vi "INitTape.vi"(5 "Settings in":T1={"max velocity"={"Value"=0.0, "Min"=0.0, "Max"=0.0, "StepSize"=0.0, "Tolerance"=0.0, "valueactual"=0.0}, "continious velocity"={"Value"=0.0, "Min"=0.0, "Max"=0.0, "StepSize"=0.0, "Tolerance"=0.0, "valueactual"=0.0}, "shake"=enum."off", "direction"=enum."left", "RedRatio"={"Value"=0.0, "Min"=0.0, "Max"=0.0, "StepSize"=0.0, "Tolerance"=0.0, "valueactual"=0.0}, "StepSize"={"Value"=0.0, "Min"=0.0, "Max"=0.0, "StepSize"=0.0, "Tolerance"=0.0, "valueactual"=0.0}, "position"={"Value"=0.0, "Min"=0.0, "Max"=0.0, "StepSize"=0.0, "Tolerance"=0.0, "valueactual"=0.0}, "velocity"={"Value"=0.0, "Min"=0.0, "Max"=0.0, "StepSize"=0.0, "Tolerance"=0.0, "valueactual"=0.0}, "Step"=enum."off", "Mode"=enum."on demand", "timeout"={"Value"=0.0, "Min"=0.0, "Max"=0.0, "StepSize"=0.0, "Tolerance"=0.0, "valueactual"=0.0}, "DelayStage"={"Value"=0.0, "Min"=0.0, "Max"=0.0, "StepSize"=0.0, "Tolerance"=0.0, "valueactual"=0.0}, "TapeMotor"=enum."off", "encoder Axis"=2, "oldpos"=0.0, "ResetEncoder"=enum."off"}, 11 "error in (no error)":errorcluster) -> (2 "Velocity (units/s) out":dbl format="%.4g", 3 "Reduction Ratio":dbl format="%.6g", 4 "VISA Refnum out":refnum<visa-resource-name>, 6 "Settings out":T1={"max velocity"={"Value"=0.0, "Min"=0.0, "Max"=0.0, "StepSize"=0.0, "Tolerance"=0.0, "valueactual"=0.0}, "continious velocity"={"Value"=0.0, "Min"=0.0, "Max"=0.0, "StepSize"=0.0, "Tolerance"=0.0, "valueactual"=0.0}, "shake"=enum."off", "direction"=enum."left", "RedRatio"={"Value"=0.0, "Min"=0.0, "Max"=0.0, "StepSize"=0.0, "Tolerance"=0.0, "valueactual"=0.0}, "StepSize"={"Value"=0.0, "Min"=0.0, "Max"=0.0, "StepSize"=0.0, "Tolerance"=0.0, "valueactual"=0.0}, "position"={"Value"=0.0, "Min"=0.0, "Max"=0.0, "StepSize"=0.0, "Tolerance"=0.0, "valueactual"=0.0}, "velocity"={"Value"=0.0, "Min"=0.0, "Max"=0.0, "StepSize"=0.0, "Tolerance"=0.0, "valueactual"=0.0}, "Step"=enum."off", "Mode"=enum."on demand", "timeout"={"Value"=0.0, "Min"=0.0, "Max"=0.0, "StepSize"=0.0, "Tolerance"=0.0, "valueactual"=0.0}, "DelayStage"={"Value"=0.0, "Min"=0.0, "Max"=0.0, "StepSize"=0.0, "Tolerance"=0.0, "valueactual"=0.0}, "TapeMotor"=enum."off", "encoder Axis"=2, "oldpos"=0.0, "ResetEncoder"=enum."off"}, 10 "downramp array":dbl[](array[numeric]), 15 "error out":errorcluster)   [LabVIEW 2011]
uses:
  TapeDrive/settings_TypDef.ctl
  shared/numericVariable_TypeDef.ctl
  shared/OnOffTypeDef.ctl
  TapeDrive/Direction_TypDef.ctl
  TapeDrive/Mode_TypDEf.ctl
  shared/CompressAndUpdate(Poly)/CompressAndUpdate(Numeric).vi
  shared/CompressAndUpdate(Poly)/CompressAndUpdate(Enum).vi
  <instrlib>/Newport ESP301/Newport ESP301.lvlib
  TapeDrive/TapeDrive.lvclass
panel:
  out "downramp array 2":dbl[](graph)
  out "Power Status":bool=TRUE
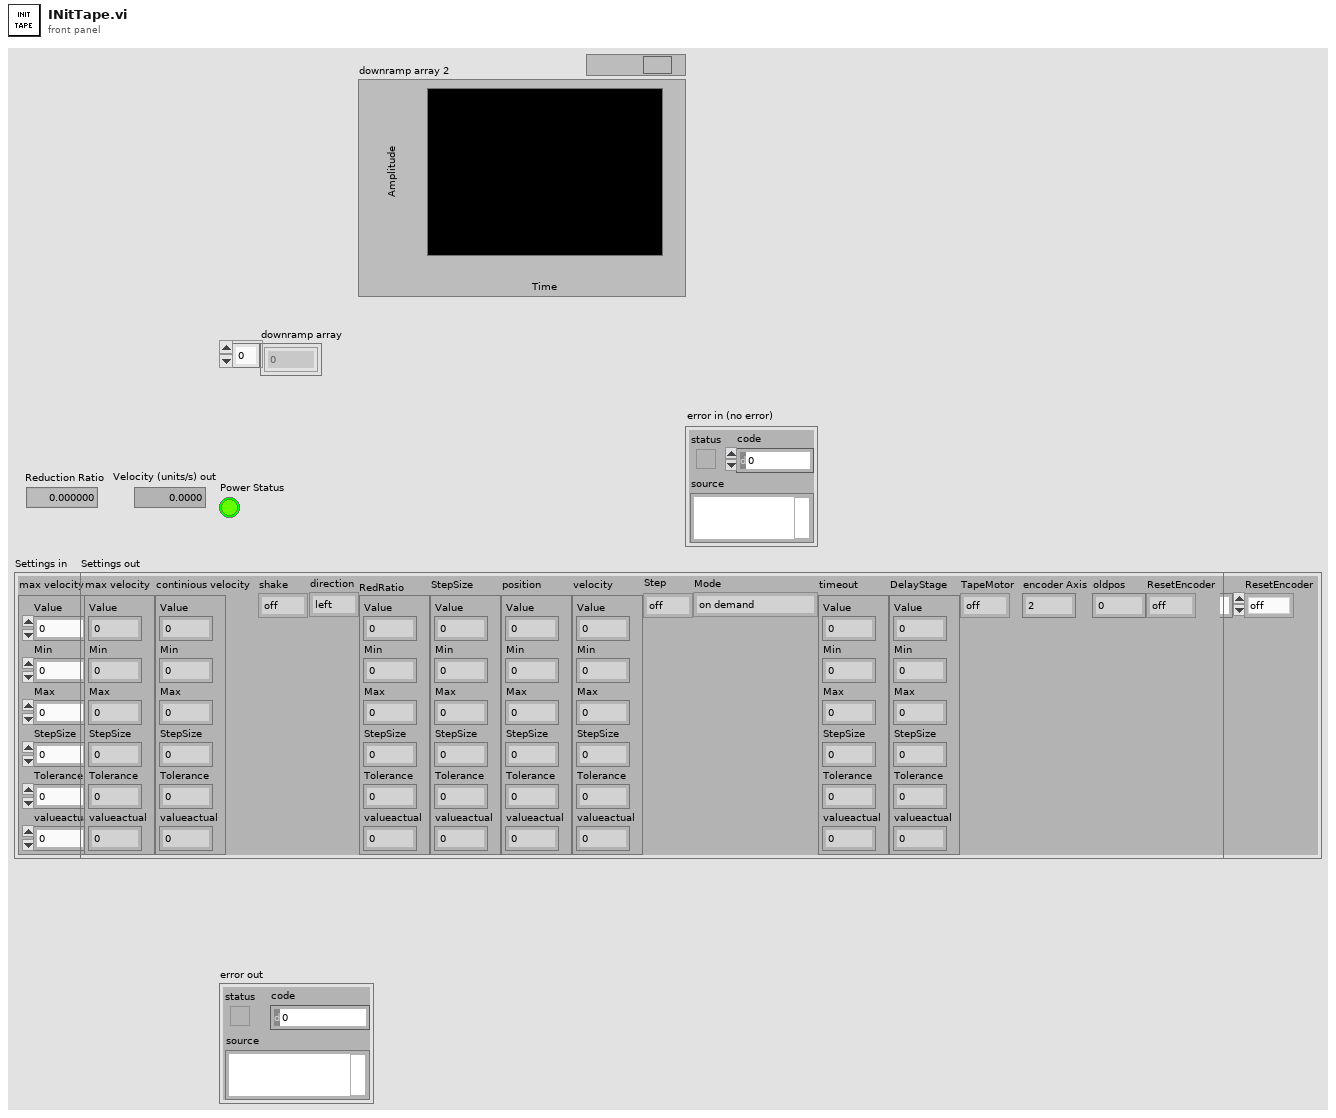
[diagram p1: front panel]
types:
  T1 = typedef "TapeDrive.lvclass/settings_TypDef.ctl" = cluster{"max velocity":T2, "continious velocity":T2, "shake":T3, "direction":T4, "RedRatio":T2, "StepSize":T2, "position":T2, "velocity":T2, "Step":T3, "Mode":T5, "timeout":T2, "DelayStage":T2, "TapeMotor":T3, "encoder Axis":i32, "oldpos":dbl, "ResetEncoder":T3}
  T2 = typedef "numericVariable_TypeDef.ctl" = cluster{"Value":dbl, "Min":dbl, "Max":dbl, "StepSize":dbl, "Tolerance":dbl, "valueactual":dbl}
  T3 = typedef "OnOffTypeDef.ctl" = enum16{"off", "on"}
  T4 = typedef "Direction_TypDef.ctl" = enum16{"left", "right"}
  T5 = typedef "Mode_TypDEf.ctl" = enum16{"on demand", "continuous", "scan"}
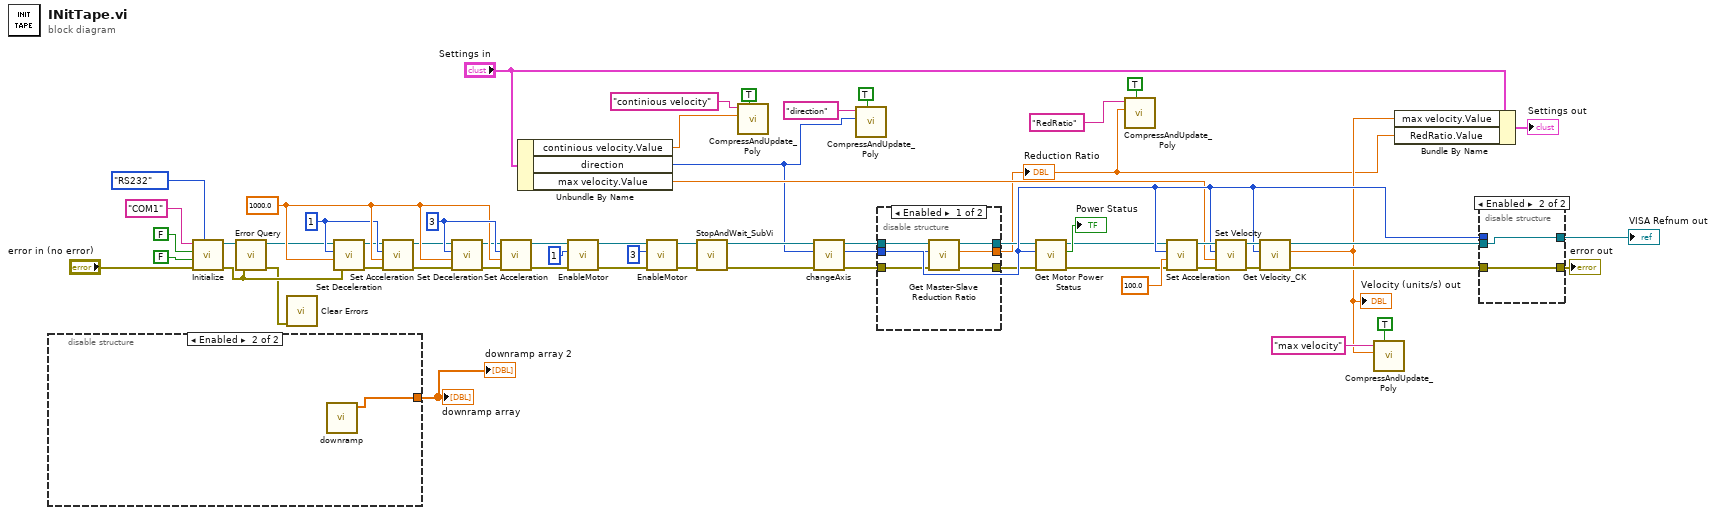
[diagram p0: block diagram]
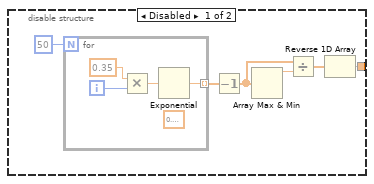
[diagram p2: hidden frame]
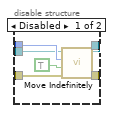
[diagram p3: hidden frame]
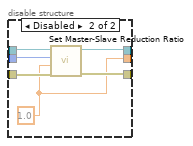
[diagram p4: hidden frame]
diagram:
  w56 = 3 ("Axis (1)")
  w48 = 1 ("Axis (1) 2")
  w55 = 1000.0 ("Acceleration (0 units/s²)")
  n1 = disable-structure shown="Enabled" {
    disable-tunnel: [w62 w72] -> w1
    frame Disabled {
      n2 = for {
        N: 50 -> [_]
        tunnel: [w71] -> w66 mode=indexing
        i -> [w70]
        (unwired) 0.30000000000000004 ("x")
        n3 = Multiply(x=0.35, y=w70) -> (x*y=w68:dbl)
        n4 = Exponential(1:w68) -> (0:w71:dbl)
      }
      n5 = Decrement(x=w66) -> (x-1=w65:dbl[])
      n6 = Array Max & Min(array=w65) -> (max value=w64:dbl)  [unwired: 3 out]
      n7 = Divide(x=w65, y=w64) -> (x/y=w63:dbl[])
      n8 = Reverse 1D Array(array=w63) -> (reversed array=w62:dbl[])
    }
    frame Enabled {
      n9 = call "downramp.vi"() -> ("downramp array"=w72:dbl[])  [unwired: 11 in]
    }
  }
  "downramp array" <- w1
  "downramp array 2" <- w1
  n10 = call <instrlib>:"Initialize.vi"("VISA resource name"="COM1" ("Settings.devport"), "ID Query (True)"=FALSE, "Reset (False)"=FALSE, "error in (no error)"="error in (no error)", "Serial Link (RS232)"=enum16{"RS232", "USB"}."RS232") -> ("VISA resource name out"=w36:refnum<visa-resource-name>, "error out"=w46:errorcluster)  [unwired: 4 in]
  n11 = call <instrlib>:"Error Query.vi"("error in (no error)"=w46, "VISA resource name"=w36) -> ("error out"=w37:errorcluster, "VISA resource name out"=w44:refnum<visa-resource-name>)  [unwired: 2 in, 2 out]
  n12 = call <vilib>:"Clear Errors.vi"("error in (no error)"=w37) -> ()  [unwired: 6 in, 1 out]
  n13 = call <instrlib>:"Set Deceleration.vi"("error in (no error)"=w46, "Deceleration (0 units/s²)"=w55, "Axis (1)"=w48, "VISA resource name"=w44) -> ("error out"=w47:errorcluster, "VISA resource name out"=w45:refnum<visa-resource-name>)  [unwired: 2 in]
  n14 = call <instrlib>:"Set Acceleration.vi"("error in (no error)"=w47, "Acceleration (0 units/s²)"=w55, "Axis (1)"=w48, "VISA resource name"=w45) -> ("error out"=w53:errorcluster, "VISA resource name out"=w51:refnum<visa-resource-name>)  [unwired: 2 in]
  n15 = call <instrlib>:"Set Deceleration.vi"("error in (no error)"=w53, "Deceleration (0 units/s²)"=w55, "Axis (1)"=w56, "VISA resource name"=w51) -> ("error out"=w49:errorcluster, "VISA resource name out"=w50:refnum<visa-resource-name>)  [unwired: 2 in]
  n16 = call <instrlib>:"Set Acceleration.vi"("error in (no error)"=w49, "Acceleration (0 units/s²)"=w55, "Axis (1)"=w56, "VISA resource name"=w50) -> ("error out"=w54:errorcluster, "VISA resource name out"=w52:refnum<visa-resource-name>)  [unwired: 2 in]
  n17 = Unbundle By Name("Settings in") -> ("continious velocity.Value"=w4:dbl, "direction"=w3:T4, "max velocity.Value"=w17:dbl)
  n18 = call "EnableMotor.vi"("error in (no error)"=w54, "Axis (1) in"=1, "VISA Refnum in"=w52) -> ("error out"=w40:errorcluster, "VISA Refnum out"=w42:refnum<visa-resource-name>)  [unwired: 7 in]
  n19 = call "EnableMotor.vi"("error in (no error)"=w40, "Axis (1) in"=3, "VISA Refnum in"=w42) -> ("error out"=w41:errorcluster, "VISA Refnum out"=w43:refnum<visa-resource-name>)  [unwired: 7 in]
  n20 = call "StopAndWait_SubVi.vi"("error in (no error)"=w41, "VISA Refnum in"=w43) -> ("error out"=w29:errorcluster, "VISA Refnum out"=w28:refnum<visa-resource-name>)  [unwired: 8 in]
  n21 = call-poly "CompressAndUpdate_Poly.vi"("force CVT update (false)"=TRUE, "Numeric"=w4, "command or variable name"="continious velocity") -> ()  [unwired: 8 in, 1 out]
  n22 = call "changeAxis.vi"("error in (no error)"=w29, "direction 2"=w3, "VISA Refnum in"=w28) -> ("error out"=w25:errorcluster, "Master"=w30:i32, "VISA Refnum out"=w31:refnum<visa-resource-name>)  [unwired: 5 in, 1 out]
  n23 = call-poly "CompressAndUpdate_Poly.vi"("force CVT update (false)"=TRUE, "enum variant"=w3, "command or variable name"="direction") -> ()  [unwired: 8 in, 1 out]
  n24 = disable-structure shown="Enabled" {
    disable-tunnel: w31 -> [w78 w84]
    disable-tunnel: w30 -> [w77 w82]
    disable-tunnel: [w76 w80] -> w26
    disable-tunnel: w25 -> [w75 w81]
    disable-tunnel: [w74 w83] -> w24
    disable-tunnel: [w73 w79] -> w10
    frame Enabled {
      n25 = call <instrlib>:"Get Master-Slave Reduction Ratio.vi"("error in (no error)"=w75, "Axis (1)"=w77, "VISA resource name"=w78) -> ("error out"=w76:errorcluster, "Reduction Ratio"=w73:dbl, "VISA resource name out"=w74:refnum<visa-resource-name>)  [unwired: 2 in]
    }
    frame Disabled {
      w79 = 1.0 ("Reduction Ratio (0)")
      n26 = call <instrlib>:"Set Master-Slave Reduction Ratio.vi"("error in (no error)"=w81, "Reduction Ratio (0)"=w79, "Axis (1)"=w82, "VISA resource name"=w84) -> ("error out"=w80:errorcluster, "VISA resource name out"=w83:refnum<visa-resource-name>)  [unwired: 2 in]
    }
  }
  "Reduction Ratio" <- w10
  n27 = call <instrlib>:"Get Motor Power Status.vi"("error in (no error)"=w26, "Axis (1)"=w30, "VISA resource name"=w24) -> ("error out"=w27:errorcluster, "Power Status"=→"Power Status":bool, "VISA resource name out"=w22:refnum<visa-resource-name>)  [unwired: 2 in]
  n28 = call-poly "CompressAndUpdate_Poly.vi"("force CVT update (false)"=TRUE, "Numeric"=w10, "command or variable name"="RedRatio") -> ()  [unwired: 8 in, 1 out]
  n29 = call <instrlib>:"Set Acceleration.vi"("error in (no error)"=w27, "Acceleration (0 units/s²)"=100.0, "Axis (1)"=w30, "VISA resource name"=w22) -> ("error out"=w60:errorcluster, "VISA resource name out"=w58:refnum<visa-resource-name>)  [unwired: 2 in]
  n30 = call <instrlib>:"Set Velocity.vi"("error in (no error)"=w60, "Velocity (units/s)"=w17, "Axis (1)"=w30, "VISA resource name"=w58) -> ("error out"=w61:errorcluster, "VISA resource name out"=w57:refnum<visa-resource-name>)  [unwired: 2 in]
  n31 = call "Get Velocity_CK.vi"("error in (no error)"=w61, "Axis (1)"=w30, "VISA resource name"=w57) -> ("error out"=w20:errorcluster, "Velocity (units/s)"=w11:dbl, "VISA resource name out"=w18:refnum<visa-resource-name>)  [unwired: 2 in]
  "Velocity (units/s) out" <- w11
  n32 = call-poly "CompressAndUpdate_Poly.vi"("force CVT update (false)"=TRUE, "Numeric"=w11, "command or variable name"="max velocity") -> ()  [unwired: 8 in, 1 out]
  n33 = Bundle By Name(cluster="Settings in", "max velocity.Value"=w11, "RedRatio.Value"=w10) -> (→"Settings out":T1)
  n34 = disable-structure shown="Enabled" {
    disable-tunnel: w30 -> [w89 _]
    disable-tunnel: [w88 w91] -> w21
    disable-tunnel: w20 -> [w87 w91]
    disable-tunnel: [w86 w92] -> w19
    disable-tunnel: w18 -> [w85 w92]
    frame Disabled {
      n35 = call <instrlib>:"Move Indefinitely.vi"("error in (no error)"=w87, "Move Direction (+)"=TRUE, "Axis (1)"=w89, "VISA resource name"=w85) -> ("error out"=w88:errorcluster, "VISA resource name out"=w86:refnum<visa-resource-name>)  [unwired: 2 in]
    }
    frame Enabled {
    }
  }
  "error out" <- w21
  "VISA Refnum out" <- w19
